vi "Write configuration.vi"(8 "error in":errorcluster, 10 "CEF Configuration":refnum<class "CEF_serializable configuration.lvclass">, 11 "DIO Channel":refnum<class "Digital IO Channel.lvclass">) -> (0 "error out":errorcluster, 3 "DIO Channel out":refnum<class "Digital IO Channel.lvclass">)   [LabVIEW 2025, in "Digital IO.lvlib" / "Digital IO Channel.lvclass"]
doc: "Copyright 2017 National Instruments Corporation\n\nLicensed under the Apache License, Version 2.0 (the \"License\"); you may not use this file except in compliance with the License. You may obtain a copy of the License at http://www.apache.org/licenses/LICENSE-2.0\nUnless required by applicable law or agreed to in writing, software distributed under the License is distributed on an \"AS IS\" BASIS, WITHOUT WARRANTIES OR CONDITIONS OF ANY KIND, either express or implied. See the License for the specific language governing permissions and limitations under the License."
uses:
  Digital IO Channel.lvclass
  Users/Public/Documents/Sandia National Labs/TSS Plugin/CEF.lvlibp/serializable configuration/CEF_serializable configuration.lvclass
  Digital IO Channel configuration/Digital IO Channel configuration.lvclass
  Digital IO Channel.lvclass/Digital IO Channel.ctl
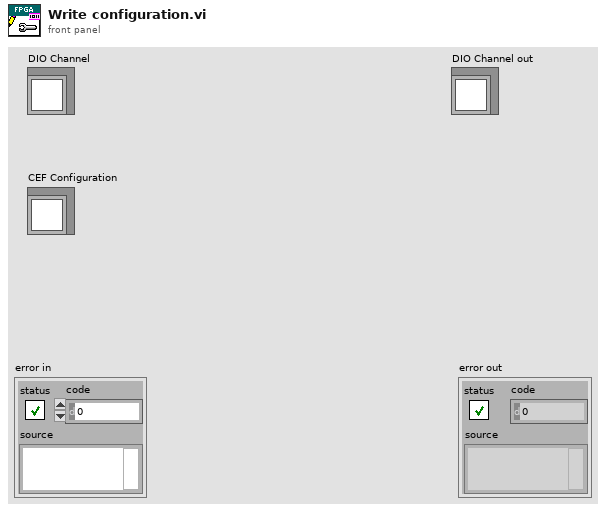
[diagram p1: front panel]
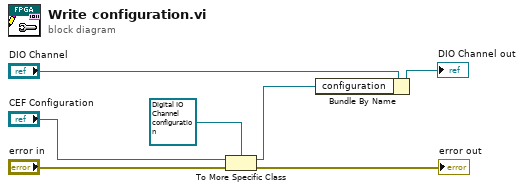
[diagram p0: block diagram]
diagram:
  n1 = To More Specific Class(target class=refnum<class "Digital IO Channel configuration.lvclass"> refnum ("configuration"), reference="CEF Configuration", error in="error in") -> (specific class reference=w4:refnum<class "Digital IO Channel configuration.lvclass">, error out=→"error out":errorcluster)
  n2 = Bundle By Name(cluster="DIO Channel", "configuration"=w4) -> (→"DIO Channel out":refnum<class "Digital IO Channel.lvclass">)
